vi "First_report.vi"() -> ()   [LabVIEW 2013]
panel:
  in  "Measurer name":string
  out "Teksti meni":path
  in  "Teksti tiedoston polku":path
  in  "Exel tiedoston polku":path
  out "Exel meni":path
  in  "stop":bool
  out "Meter":dbl(knob) scale=0.0..10.0
  in  "Knob":dbl(knob) scale=0.0..10.0
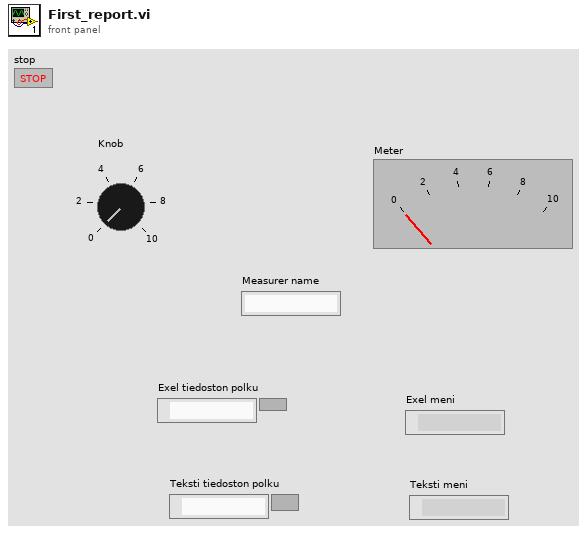
[diagram p1: front panel]
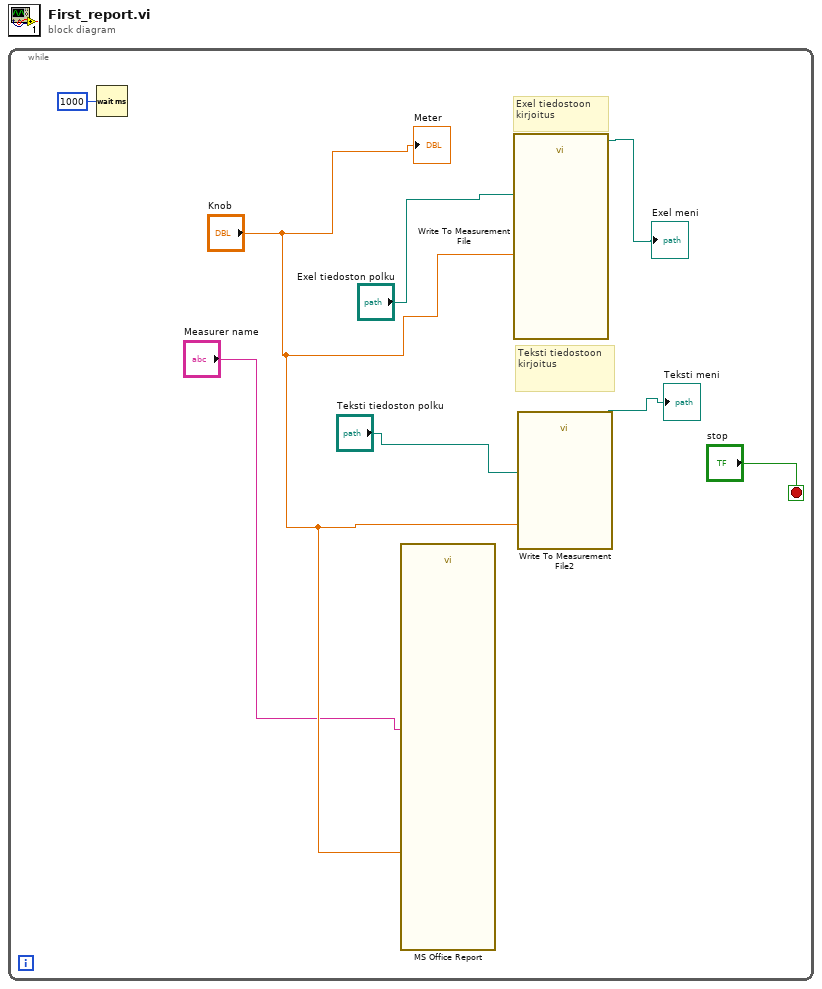
[diagram p0: block diagram]
diagram:
  n1 = while {
    stop <- "stop" stop-if-true
    # "Teksti tiedostoon kirjoitus"
    # "Exel tiedostoon kirjoitus"
    n2 = Wait (ms)(milliseconds to wait=u32 1000) -> ()  [unwired: 1 out]
    n3 = call "MS Office Report"("Author_Name"="Measurer name", "Table1_Data_Input"="Knob") -> ()  [unwired: 25 in, 1 out]
    n4 = call "Write To Measurement File"("Signals"="Knob", "Filename"="Exel tiedoston polku") -> ("Filename Out"=→"Exel meni":path)  [unwired: 15 in, 2 out]
    n5 = call "Write To Measurement File2"("Signals"="Knob", "Filename"="Teksti tiedoston polku") -> ("Filename Out"=→"Teksti meni":path)  [unwired: 15 in, 2 out]
    "Meter" <- "Knob"
  }
